vi "parseNumberArray.vi"(8 "error in (no error)":errorcluster, 10 "commandData":string, 11 "CoolerSerialCommand in":refnum<class "CoolerSerialCommand.lvclass">) -> (0 "error out":errorcluster, 2 "NumberArray":u16[](array[numeric]), 3 "CoolerSerialCommand out":refnum<class "CoolerSerialCommand.lvclass">)   [LabVIEW 2016, in "CoolerSerialCommand.lvclass"]
uses:
  CoolerSerialCommand.lvclass
panel:
  out "substring":string
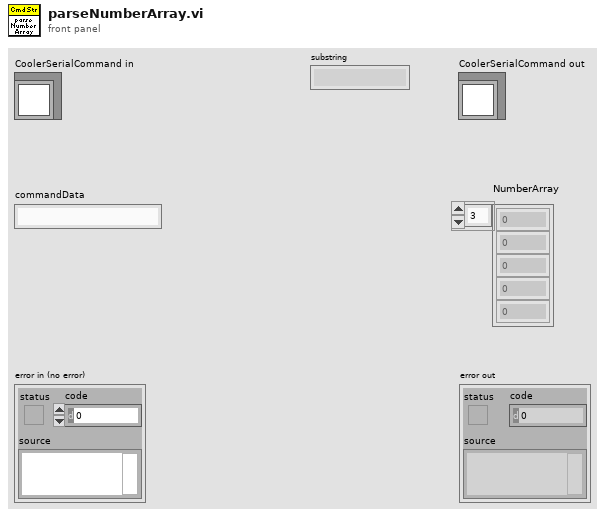
[diagram p1: front panel]
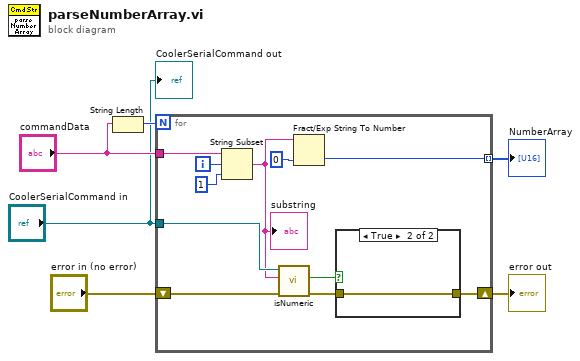
[diagram p0: block diagram]
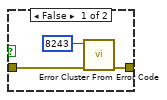
[diagram p2: hidden frame]
diagram:
  n1 = String Length(string="commandData") -> (length=w6:i32)
  n2 = for {
    N: w6 -> [_]
    tunnel: "commandData" -> [w15]
    tunnel: [w14] -> w4 mode=indexing
    tunnel: "CoolerSerialCommand in" -> [w11]
    shift-right: [w7] -> w1
    shift-left: "error in (no error)" -> [w12]
    i -> [w13]
    n3 = String Subset(string=w15, offset (0)=w13, length (rest)=1 ("length (rest)")) -> (substring=w10:string)
    "substring" <- w10
    n4 = call "isNumeric"("error in (no error)"=w12, "numberString"=w10, "CoolerSerialCommand in"=w11) -> ("error out"=w8:errorcluster, "isNumeric?"=w9:bool)  [unwired: 6 in, 1 out]
    n5 = Fract/Exp String To Number(string=w10, default (0 dbl)=u16 0 ("value")) -> (number=w14:u16)  [unwired: 2 in, 1 out]
    n6 = case shown="True" w9 {
      tunnel: [w19 w21] -> w7
      tunnel: w8 -> [w20 w21]
      frame False {
        n7 = call <vilib>:"Error Cluster From Error Code.vi"("error in (no error)"=w20, "error code (0)"=8243) -> ("error out"=w19:errorcluster)  [unwired: 7 in]
      }
      frame True {
      }
    }
  }
  "error out" <- w1
  "NumberArray" <- w4
  "CoolerSerialCommand out" <- "CoolerSerialCommand in"
